vi "MultiFPGAAPUTest.vi"() -> ()   [LabVIEW 2015]
uses:
  Version Token.ctl
  APU/Settings.ctl
  APU/Input.ctl
  APU/Output.ctl
  APU/Shared Settings.ctl
  <vilib>/Platform/TimedLoop/XDataNode/timing_clust.ctl
  <vilib>/Platform/TimedLoop/XDataNode/nitl_modes.ctl
  <vilib>/Platform/TimedLoop/XDataNode/wakeup.ctl
  <vilib>/rvi/Emulation/niFpgaSctlEmulationGetInTimedLoop.vi
  <vilib>/rvi/Emulation/niFpgaEmulationReportErrorSimple.vi
  <vilib>/rvi/Emulation/niFpgaGetClockAttributes.vi
  <vilib>/rvi/Emulation/niFpgaCriticalErrorInLSC.vi
  <vilib>/Platform/TimedLoop/XDataNode/XDataNode.xnode
  <vilib>/Platform/TimedLoop/XDataNode/XDNodeRunTimeDep.lvlib
  APU/APU.lvlib
  Engine Simulation Toolkit.lvlib
panel:
  in  "master.apu 1":bool
  in  "send trigger.apu 1":bool
  in  "trigger line.apu 1":refnum<k21>="PXI_Trig0"
  in  "shared settings.apu 1":T1 {"start" format="%#.15g"}
  in  "go.apu 1":bool
  out "output.apu 1":T2 caption="output"
  in  "input.apu 1":T3={"desired speed"=0.0, "reset"=TRUE} caption="input"
  in  "settings.apu 1":T4 caption="settings"
  in  "est.version":T5
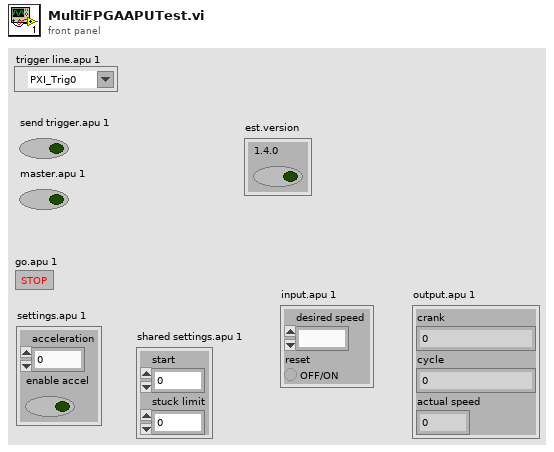
[diagram p1: front panel]
types:
  T1 = typedef "Engine Simulation Toolkit.lvlib/APU.lvlib/Shared Settings.ctl" = cluster{"start":fxp<+,17,17>, "stuck limit":fxp<+,18,18>}
  T2 = typedef "Engine Simulation Toolkit.lvlib/APU.lvlib/Output.ctl" = cluster{"crank":u16, "cycle":u16, "actual speed":fxp<+/-,23,2>}
  T3 = typedef "Engine Simulation Toolkit.lvlib/APU.lvlib/Input.ctl" = cluster{"desired speed":fxp<+/-,23,2>, "reset":bool}
  T4 = typedef "Engine Simulation Toolkit.lvlib/APU.lvlib/Settings.ctl" = cluster{"acceleration":fxp<+,18,-20>, "enable accel":bool}
  T5 = typedef "Engine Simulation Toolkit.lvlib/Version Token.ctl" = cluster{"1.4.0":bool}
  T6 = typedef "XDNodeRunTimeDep.lvlib/timing_clust.ctl" = cluster{"Expected End [f-1]":u64, "Actual End [f-1]":u64, "Finished Late? [f-1]":bool, "Expected End [i-1]":u64, "Actual End [i-1]":u64, "Finished Late? [i-1]":bool, "Expected Start [i]":u64, "Actual Start [i]":u64, "Expected Start [f]":u64, "Actual Start [f]":u64, "Source Name":string, "Structure Name":string, "Period":i64, "Deadline":i64, "Offset":i64, "Start":i64, "Priority":i32, "Timeout":i32, "Mode":T7, "Wakeup Reason":T8, "Error":errorcluster, "Source Type":string, "Secondary Source Type":string, "Global End Time":u64, "Global Start Time":u64, "Frame Duration":u64, "Iteration Duration":u64, "Assigned CPU":i32, "I/O Scan Engine Mode":u32}
  T7 = typedef "XDNodeRunTimeDep.lvlib/nitl_modes.ctl" = enum32{"No Change", "Process missed periods, maintain original phase", "Discard missed periods, maintain original phase", "Process missed periods, ignore original phase", "Discard missed periods, ignore original phase"}
  T8 = typedef "XDNodeRunTimeDep.lvlib/wakeup.ctl" = enum32{"Normal", "Aborted", "Asynchronous wakeup", "Timing source error", "Timed loop error", "Timeout"}
  T9 = typedef "Engine Simulation Toolkit.lvlib/APU.lvlib/Register Bus.ctl" = cluster{"Speed":refnum<k21>, "Crank Angle":refnum<k21>, "Cycle Angle":refnum<k21>, "Crank Count":refnum<k21>, "Cycle Count":refnum<k21>, "1.25 MHz Counter":refnum<k21>, "Crank Rollover":refnum<k21>, "Cycle Rollover":refnum<k21>, "shared settings":T1}
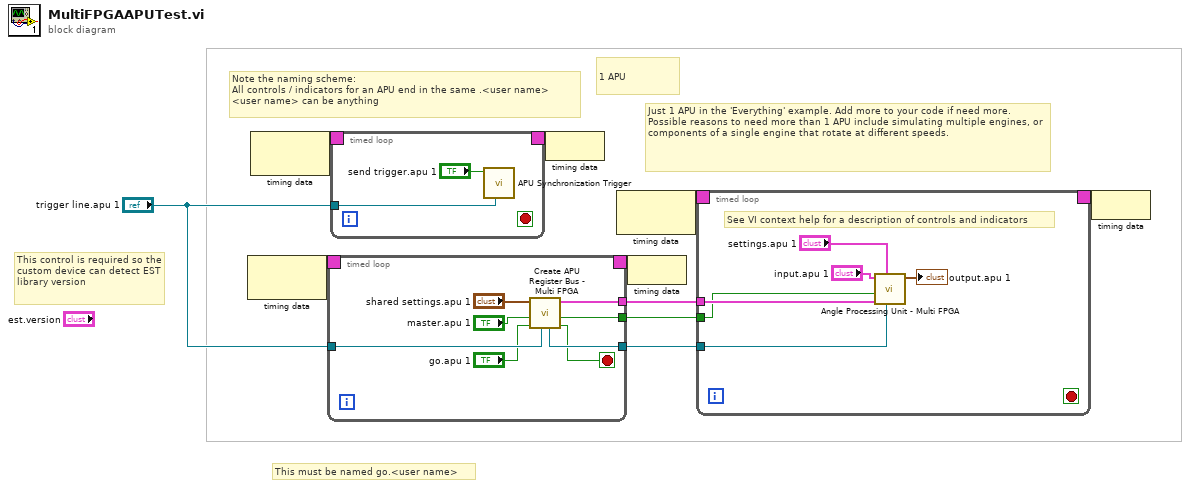
[diagram p0: block diagram]
diagram:
  # "This must be named go.<user name>"
  # "1 APU"
  # "Note the naming scheme: \nAll controls / indicators for an APU end in the same .<user name>\n<user name> can be anything"
  # "Just 1 APU in the 'Everything' example. Add more to your code if need more. Possible reasons to need more than 1 APU include simulating multiple engines, or components of a single engine that rotate at different speeds."
  # "This control is required so the custom device can detect EST library version"
  n1 = node-c288() -> (w8:T6)  [unwired: 1 in]
  n2 = node-c288() -> (w4:T6)  [unwired: 1 in]
  n3 = timed-loop {
    timing: w8 -> [_]
    timing-out: [_] -> w7
    tunnel: [w17] -> w6
    tunnel: [w16] -> w5
    tunnel: "trigger line.apu 1" -> [w15]
    tunnel: [w12] -> w1
    stop <- w11 stop-if-true
    n4 = call "Create APU Register Bus - Multi FPGA.vi"("trigger line.<user name>"=w15, "go.<user name>"="go.apu 1", "master.<user name>"="master.apu 1", "shared settings.<user name>"="shared settings.apu 1") -> ("go?"=w11:bool, "master?"=w12:bool, "register bus"=w17:T9, "trigger line"=w16:refnum<k21>)  [unwired: 4 in]
  }
  n5 = timed-loop {
    timing: w4 -> [_]
    timing-out: [_] -> w3
    tunnel: "trigger line.apu 1" -> [w21]
    stop <- _ stop-if-true
    n6 = call "APU Synchronization Trigger.vi"("trigger line.<user name>"=w21, "send trigger.<user name>"="send trigger.apu 1") -> ()  [unwired: 10 in]
  }
  n7 = node-c288(w3) -> ()
  n8 = node-c288() -> (w10:T6)  [unwired: 1 in]
  n9 = node-c288(w7) -> ()
  n10 = timed-loop {
    timing: w10 -> [_]
    timing-out: [_] -> w9
    tunnel: w6 -> [w27]
    tunnel: w5 -> [w26]
    tunnel: w1 -> [w25]
    stop <- _ stop-if-true
    # "See VI context help for a description of controls and indicators"
    n11 = call "Angle Processing Unit - Multi FPGA.vi"("trigger line.<user name>"=w26, "settings.<user name>"="settings.apu 1", "register bus"=w27, "master"=w25, "input.<user name>"="input.apu 1") -> ("output.<user name>"=→"output.apu 1":T2)  [unwired: 6 in]
  }
  n12 = node-c288(w9) -> ()
